vi "string_concat.vi"(6 "Step di frequenza (Hz)":string, 7 "Ampiezza (Vpp)":string, 9 "f_stop (Hz)":string, 10 "f_start (Hz)":string, 11 "Password":string) -> (3 "Comando concatenato":string)   [LabVIEW 2021]
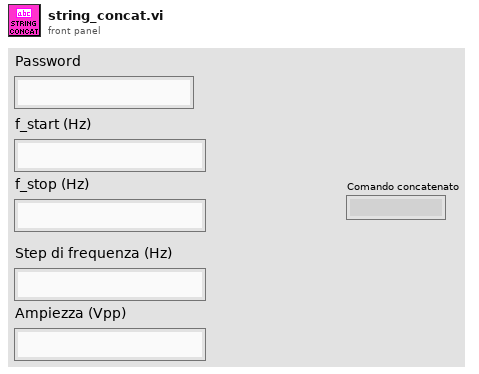
[diagram p1: front panel]
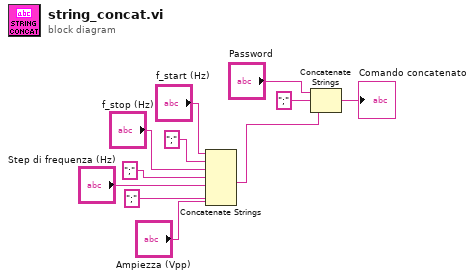
[diagram p0: block diagram]
diagram:
  n1 = Concatenate Strings("f_start (Hz)", ";" ("string"), "f_stop (Hz)", ";" ("string"), "Step di frequenza (Hz)", ";" ("string"), "Ampiezza (Vpp)") -> (w7:string)
  n2 = Concatenate Strings("Password", ";" ("string"), w7) -> (→"Comando concatenato":string)
